vi "RecordingFileName.vi"   [LabVIEW 2018, in "OXYGEN.lvlib"]
uses:
  OXYGEN.lvlib
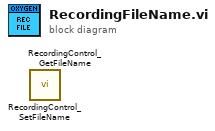
[diagram p0: block diagram]
diagram:
  n1 = call "RecordingControl_SetFileName.vi"() -> ()  [unwired: 9 in, 3 out]
  n2 = call "RecordingControl_GetFileName.vi"() -> ()  [unwired: 8 in, 4 out]
